vi "FTW-Actor-Destroy.vi"(0 "FTW Actor":refnum<class "FTW-Actor.lvclass">, 11 "error in":errorcluster) -> (15 "error out":errorcluster)   [LabVIEW 2014, in "FTW-Actor.lvclass"]
uses:
  FTW-Actor.lvclass
  Sequencer/FTW-Sequencer.lvclass
  Reference/FTW-ActorReference.lvclass
  Messaging/FTW-Actor-Broker.lvclass
panel:
  # "Inputs"
  # "Outputs"
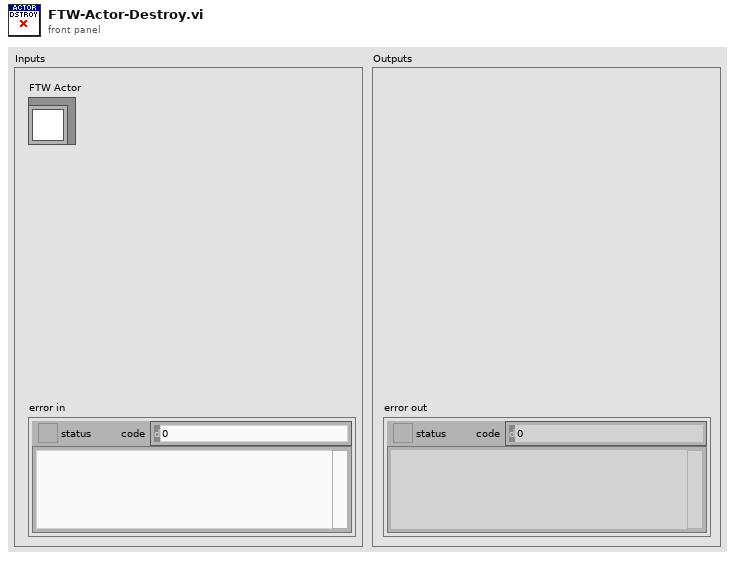
[diagram p1: front panel]
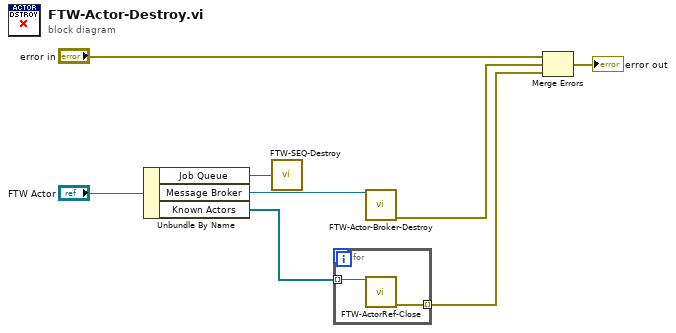
[diagram p0: block diagram]
diagram:
  n1 = Unbundle By Name("FTW Actor") -> ("Job Queue"=w5:refnum<class "FTW-Sequencer.lvclass">, "Message Broker"=w2:refnum<class "FTW-Actor-Broker.lvclass">, "Known Actors"=w4:refnum<class "FTW-ActorReference.lvclass">[])
  n2 = call "FTW-SEQ-Destroy.vi"("Sequencer"=w5) -> ()  [unwired: 1 in]
  n3 = for {
    tunnel: w4 -> [w10] mode=indexing
    tunnel: [w9] -> w3 mode=indexing
    n4 = call "FTW-ActorRef-Close.vi"("FTW Actor Reference"=w10) -> ("error out"=w9:errorcluster)  [unwired: 14 in]
  }
  n5 = call "FTW-Actor-Broker-Destroy.vi"("FTW Message Broker"=w2) -> ("error out"=w1:errorcluster)  [unwired: 14 in]
  n6 = Merge Errors("error in", w1, w3) -> (→"error out":errorcluster)
